vi "RT_MasterLoopvi.vi"   [LabVIEW 2016]
uses:
  Shared Libraries/VN100/TypeDef/AsyncMode.ctl
  <vilib>/FPGAPlugInAG/PXI-7842R/niLvFpga_Open_PXI-7842R.vi
  <vilib>/rvi/interface/common/dynamic/niFpgaDynamicAddResources.vi
  <vilib>/rvi/interface/nirviOpenFPGA/nirviOpenFPGA.xnode
  FPGA Bitfiles/CAlex2_FPGATarget_MotorControl_+dy1qhm6Ymw.lvbitx
  Shared Libraries/VN100/VN100.lvclass
panel:
  # "This VI can only be stopped by pressing the stop button on the control interface VI"
types:
  T1 = typedef "VN100.lvclass/AsyncMode.ctl" = enum16{"VNYPR", "VNYMR"}
  T2 = typedef "LowLvControl Cluster.ctl" = cluster{"MotorCtrl":refnum<class "MotorControl.lvclass">, "FPGA Ref":refnum<k20>, "AI Task":refnum<k21>, "Encoder Tasks":refnum<k21>[]}
  T3 = typedef "HighLvControl Cluster.ctl" = cluster{"CAlex2 out":refnum<class "CAlex2.lvclass">, "ForceField":refnum<class "ForceField.lvclass">}
  T4 = typedef "Logger Cluster.ctl" = cluster{"Data Logger out":refnum<class "Data Logger.lvclass">, "SyncIn":refnum<k21>, "SyncOut":refnum<k21>}
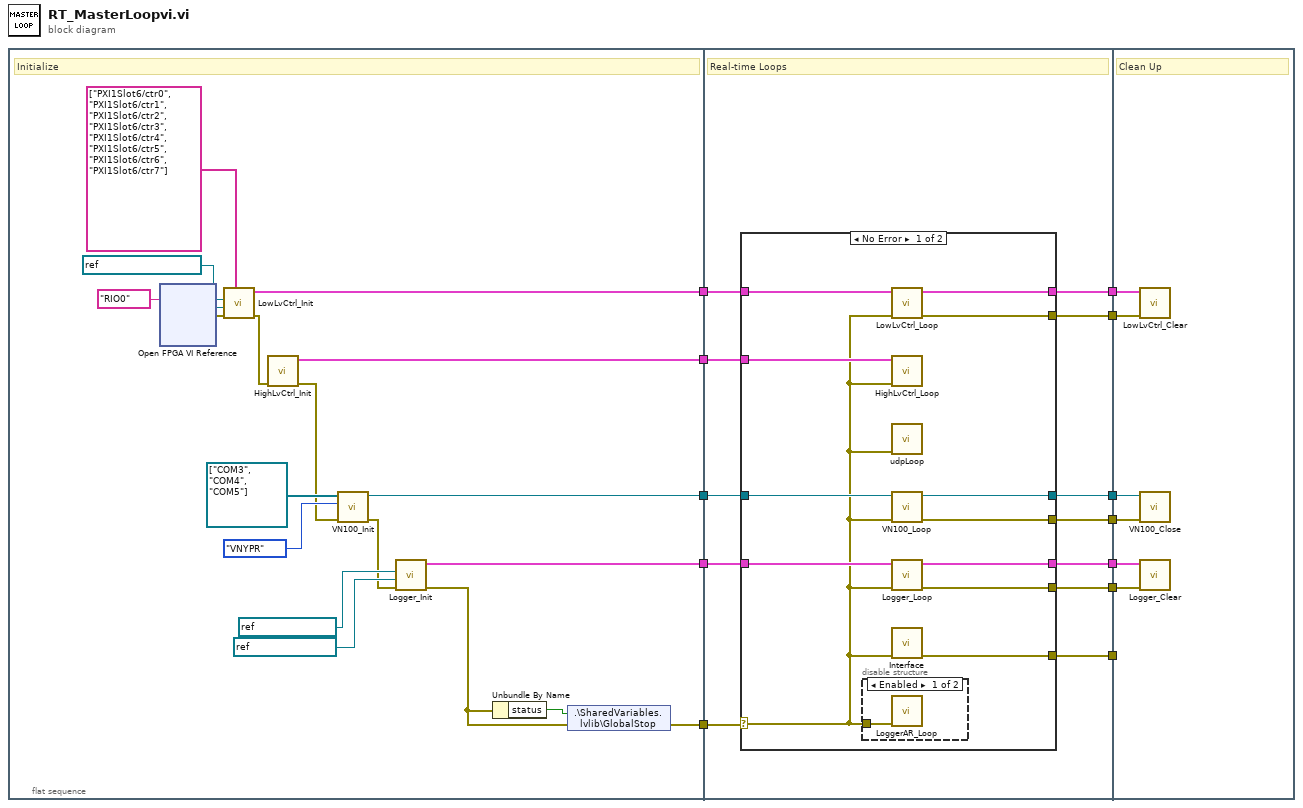
[diagram p0: block diagram]
diagram:
  n1 = flat-sequence {
    tunnel: [w13] -> w12
    tunnel: [w31] -> w11
    tunnel: [w29] -> w7
    tunnel: [w22] -> w6
    tunnel: [w21] -> w5
    tunnel: w12 -> [w43]
    tunnel: w11 -> [w42]
    tunnel: [w41] -> w10
    tunnel: [w40] -> w9
    tunnel: [w39] -> w8
    tunnel: w7 -> [w38]
    tunnel: w6 -> [w37]
    tunnel: w5 -> [w36]
    tunnel: [w35] -> w4
    tunnel: [w34] -> w3
    tunnel: [w33] -> w2
    tunnel: [w32] -> w1
    tunnel: w10 -> [w66]
    tunnel: w9 -> [w65]
    tunnel: w8 -> [_]
    tunnel: w4 -> [w62]
    tunnel: w3 -> [w64]
    tunnel: w2 -> [w63]
    tunnel: w1 -> [w61]
    frame #0 {
      # "Initialize"
      n2 = xnode "Open FPGA VI Reference"("resource name"=tag "RIO0") -> ("FPGA VI Reference Out"=w25:refnum<k20>, "error out"=w24:errorcluster)  [unwired: 1 in]
      n3 = call "LowLvCtrl_Init.vi"("Encoder Tasks In"=tag[] ["PXI1Slot6/ctr0", "PXI1Slot6/ctr1", "PXI1Slot6/ctr2", "PXI1Slot6/ctr3", "PXI1Slot6/ctr4", "PXI1Slot6/ctr5", "PXI1Slot6/ctr6", "PXI1Slot6/ctr7"], "error in (no error)"=w24, "Analog Task In"=refnum<k21> "LoadCells_FSR_AI", "FPGA VI Reference In"=w25) -> ("error out"=w30:errorcluster, "LowLvControl"=w13:T2)  [unwired: 6 in]
      n4 = call "HighLvCtrl_Init.vi"("error in (no error)"=w30) -> ("error out"=w15:errorcluster, "HighLvClasses"=w31:T3)  [unwired: 9 in]
      n5 = call "VN100_Init.vi"("error in (no error)"=w15, "AsyncMode(VNYPR)"=AsyncMode."VNYPR" ("AsyncMode"), "Serial Ports"=refnum<visa-resource-name>[] ["COM3", "COM4", "COM5"]) -> ("error out"=w18:errorcluster, "VN100 out"=w22:refnum<class "VN100.lvclass">)  [unwired: 7 in]
      n6 = call "Logger_Init.vi"("error in (no error)"=w18, "SyncOut"=refnum<k21> "SyncOut_EMG" ("SyncOut_EMG"), "SyncIn"=refnum<k21> "SyncIn_Vicon" ("SyncOut_EMG")) -> ("error out"=w17:errorcluster, "Logger Loop Cluster"=w21:T4)  [unwired: 7 in]
      n7 = Unbundle By Name(w17) -> ("status"=w28:bool)
      n8 = shared-variable ".\\SharedVariables.lvlib\\GlobalStop"(w28, error in=w17) -> (error out=w29:errorcluster)
    }
    frame #1 {
      # "Real-time Loops"
      n9 = case shown="No Error" w38 {
        selector: w38 -> [w45 w58]
        tunnel: w43 -> [w48 w59]
        tunnel: w42 -> [w51 _]
        tunnel: [w55 w60] -> w41
        tunnel: [w54 w58] -> w40
        tunnel: [w53 w58] -> w39
        tunnel: w37 -> [w52 w60]
        tunnel: [w50 w58] -> w35
        tunnel: w36 -> [w49 w57]
        tunnel: [w47 w59] -> w34
        tunnel: [w46 w58] -> w33
        tunnel: [w44 w57] -> w32
        frame No Error {
          n10 = disable-structure shown="Enabled" {
            disable-tunnel: w45 -> [w56 _]
            frame Enabled {
              n11 = call "LoggerAR_Loop.vi"("error in (no error)"=w56) -> ()  [unwired: 10 in, 1 out]
            }
            frame Disabled {
            }
          }
          n12 = call "LowLvCtrl_Loop.vi"("error in (no error)"=w45, "LowLvControl in"=w48) -> ("error out"=w46:errorcluster, "LowLvControl out"=w47:T2)  [unwired: 8 in]
          n13 = call "HighLvCtrl_Loop.vi"("error in (no error)"=w45, "HighLvClasses"=w51) -> ()  [unwired: 9 in, 1 out]
          n14 = call "udpLoop.vi"("error in (no error)"=w45) -> ()  [unwired: 10 in, 1 out]
          n15 = call "VN100_Loop.vi"("error in (no error)"=w45, "VN100 In"=w52) -> ("error out"=w54:errorcluster, "VN100 Out"=w55:refnum<class "VN100.lvclass">)  [unwired: 8 in]
          n16 = call "Logger_Loop.vi"("error in (no error)"=w45, "Logger Loop Cluster in"=w49) -> ("error out"=w50:errorcluster, "Logger Cluster out"=w44:T4)  [unwired: 8 in]
          n17 = call "Interface.vi"("error in (no error)"=w45) -> ("error out"=w53:errorcluster)  [unwired: 10 in]
        }
        frame Error {
        }
      }
    }
    frame #2 {
      # "Clean Up"
      n18 = call "LowLvCtrl_Clear.vi"("error in (no error)"=w63, "LowLvControl"=w64) -> ()  [unwired: 9 in, 1 out]
      n19 = call "VN100_Close.vi"("error in (no error)"=w65, "VN100 in"=w66) -> ()  [unwired: 9 in, 1 out]
      n20 = call "Logger_Clear.vi"("error in (no error)"=w62, "Logger Loop Cluster"=w61) -> ()  [unwired: 9 in, 1 out]
    }
  }
